vi "Read SPI.vi"(8 "error in (no error)":errorcluster, 9 "Len":u8, 10 "Bus":u8, 11 "VISA resource name in":refnum<visa-resource-name>) -> (0 "error out":errorcluster, 1 "Data":string, 3 "VISA resource name":refnum<visa-resource-name>)   [LabVIEW 2023, in "CTI-Visa.lvlib"]
uses:
  CTI-Visa.lvlib
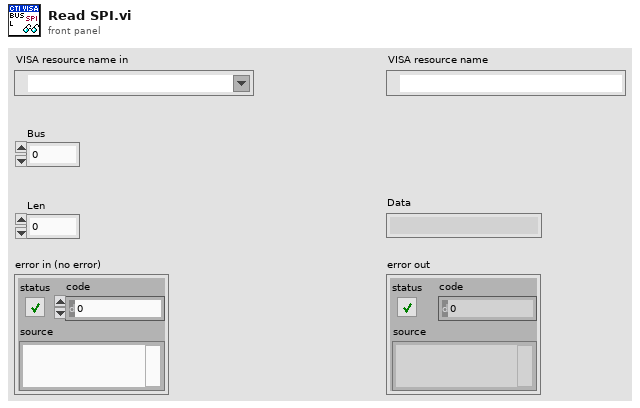
[diagram p1: front panel]
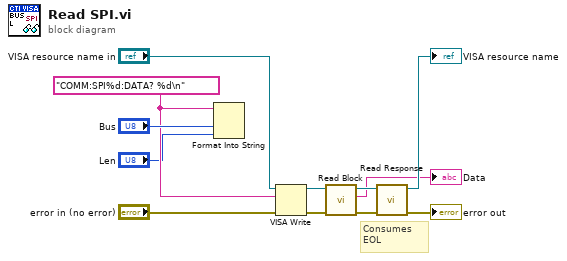
[diagram p0: block diagram]
diagram:
  w9 = "COMM:SPI%d:DATA? %d\n" ("format string")
  # "Consumes EOL"
  n1 = Format Into String(format string=w9, "Bus", "Len") -> ()  [unwired: 2 in, 2 out]
  n2 = VISA Write(VISA resource name="VISA resource name in", write buffer=w9, error in (no error)="error in (no error)") -> (VISA resource name out=w7:refnum<visa-resource-name>, error out=w8:errorcluster)  [unwired: 1 out]
  n3 = call "Read Block.vi"("error in (no error)"=w8, "VISA resource name in"=w7) -> ("error out"=w6:errorcluster, "Block Data"=→"Data":string, "VISA resource name"=w5:refnum<visa-resource-name>)  [unwired: 7 in]
  n4 = call "Read Response.vi"("error in (no error)"=w6, "VISA resource name in"=w5) -> ("error out"=→"error out":errorcluster, "VISA resource name"=→"VISA resource name":refnum<visa-resource-name>)  [unwired: 7 in, 1 out]
